vi "StripCommand.vi"(11 "Command":string) -> (3 "Stripped Command":string)   [LabVIEW 2012, in "Omega-CSi32.lvlib"]
uses:
  Omega-CSi32.lvlib
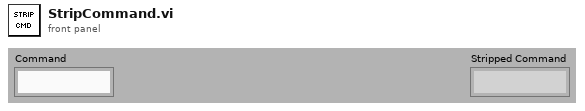
[diagram p1: front panel]
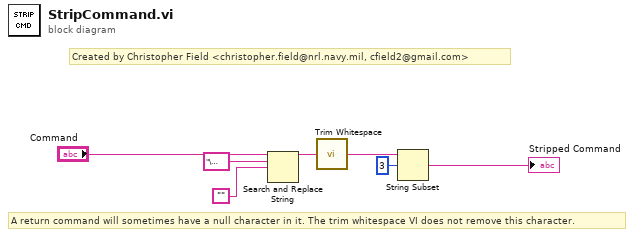
[diagram p0: block diagram]
diagram:
  # "Created by Christopher Field <christopher.field@nrl.navy.mil, cfield2@gmail.com>"
  # "A return command will sometimes have a null character in it. The trim whitespace VI does not remove this character."
  n1 = Search and Replace String(input string="Command", search string="\u0000", replace string="") -> (result string=w2:string)  [unwired: 5 in, 3 out]
  n2 = call <vilib>:"Trim Whitespace.vi"("string"=w2) -> ("trimmed string"=w1:string)  [unwired: 1 in]
  n3 = String Subset(string=w1, offset (0)=3) -> (substring=→"Stripped Command":string)  [unwired: 1 in]
